vi "Test Override Inherited Test Name.vi"(8 "error in (no error)":errorcluster, 11 "Test Case In":refnum<class "Inheritance Test.lvclass">) -> (0 "error out":errorcluster, 3 "Test Case Out":refnum<class "Inheritance Test.lvclass">)   [LabVIEW 2020, in "Inheritance Test.lvclass"]
uses:
  Inheritance Test.lvclass
  C:/Program Files (x86)/National Instruments/LabVIEW 2020/vi.lib/Astemes/LUnit/Test Case.lvclass
  source/LUnit Inheriting Test Case/LUnit Inheriting Test Case.lvclass
  <vilib>/Astemes/LUnit/Test Case.lvclass/Test Case.ctl
  <vilib>/Astemes/LUnit/Append Fail Result.vi
  <vilib>/Astemes/LUnit/Append Pass Result.vi
  <vilib>/Astemes/LUnit/Run In UI.vi
  <vilib>/Utility/error.llb/Clear Errors.vi
  <vilib>/Astemes/LUnit/Test Suite.lvclass
  C:/Program Files (x86)/National Instruments/LabVIEW 2020/vi.lib/Astemes/LUnit/LUnit Runnable.lvclass
  Inheritance Test.lvclass/Inheritance Test.ctl
  <vilib>/Astemes/LUnit/Test Case.lvclass
  <vilib>/Astemes/LUnit/LUnit Runnable.lvclass
  C:/git/astemes-lunit-test-inheritance/tests/Inheritance Test/Inheritance Test.lvclass
  C:/Program Files (x86)/National Instruments/LabVIEW 2020/vi.lib/Astemes/LUnit/Test Suite.lvclass
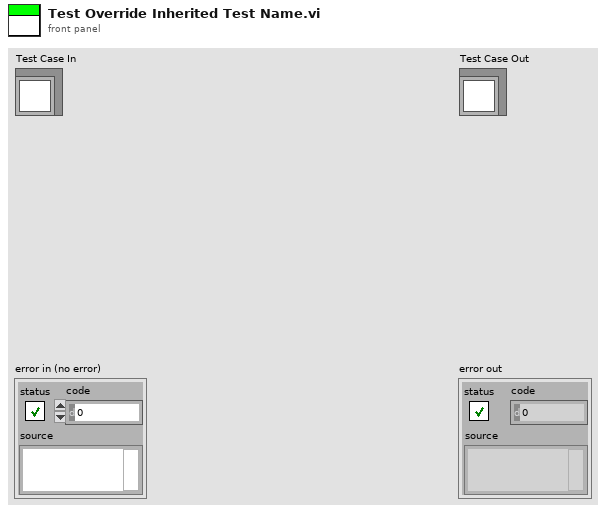
[diagram p1: front panel]
types:
  T1 = enum16{"", "Passed", "Failed", "Error", "Skipped", "Setup Error", "Broken", "Teardown Error"}
  T2 = cluster{"Name":string, "Message":string, "Description":string, "Status":enum16{"", "Passed", "Failed", "Error", "Skipped", "Setup Error", "Broken", "Teardown Error"}, "Result Type":enum16{"Test Case", "Test Suite", "Test Run", "Pass", "Fail", "Skip", "Pass if", "Fail if", "Pass if Error", "Fail if Error", "Pass if Equal", "Fail if Equal"}, "Execution Time":dbl}[]
  T3 = enum16{"Test Case", "Test Suite", "Test Run", "Pass", "Fail", "Skip", "Pass if", "Fail if", "Pass if Error", "Fail if Error", "Pass if Equal", "Fail if Equal"}
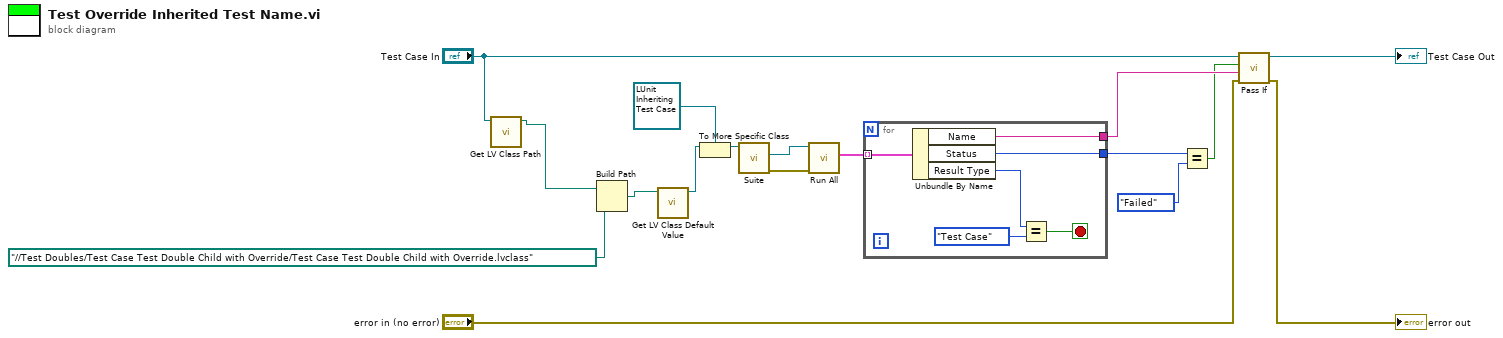
[diagram p0: block diagram]
diagram:
  n1 = call <vilib>:"Get LV Class Path.vi"("object"="Test Case In") -> ("class path"=w6:path)  [unwired: 9 in, 1 out]
  n2 = Build Path(base path=w6, name or relative path=path "../../Test Doubles/Test Case Test Double Child with Override/Test Case Test Double Child with Override.lvclass" ("Relative Path from 1 to 2")) -> (appended path=w5:path)
  n3 = call <vilib>:"Get LV Class Default Value.vi"("class path"=w5) -> ("object"=w4:refnum<class>)  [unwired: 9 in, 1 out]
  n4 = To More Specific Class(target class=refnum<class "LUnit Inheriting Test Case.lvclass"> refnum ("LUnit Test Case out"), reference=w4) -> (specific class reference=w3:refnum<class "LUnit Inheriting Test Case.lvclass">)  [unwired: 1 in, 1 out]
  n5 = call-dynamic "Suite.vi"("LUnit Test Case in"=w3) -> ("error out"=w14:errorcluster, "LUnit Test Suite Out"=w8:refnum<class "Test Suite.lvclass">)  [unwired: 8 in, 1 out]
  n6 = call <vilib>:"Run All.vi"("error in (no error)"=w14, "Runnable In"=w8) -> ("Results"=w13:T2)  [unwired: 8 in, 1 out]
  n7 = for {
    tunnel: w13 -> [w23] mode=indexing
    tunnel: [w19] -> w12
    tunnel: [w18] -> w11
    stop <- w20 stop-if-true
    n8 = Unbundle By Name(w23) -> ("Name"=w19:string, "Status"=w18:T1, "Result Type"=w22:T3)
    n9 = Equal?(x=w22, y=T3."Test Case") -> (x = y?=w20:bool)
  }
  n10 = Equal?(x=w11, y=T1."Failed") -> (x = y?=w9:bool)
  n11 = call <vilib>:"Pass If.vi"("error in (no error)"="error in (no error)", "Message"=w12, "Pass?"=w9, "LUnit Test Case In"="Test Case In") -> ("error out"=→"error out":errorcluster, "LUnit Test Case Out"=→"Test Case Out":refnum<class "Inheritance Test.lvclass">)  [unwired: 6 in]
